vi "Left Find Data String (SubVI).vi"(11 "Sampled Data":string) -> (3 "Data String":string)   [LabVIEW 2015]
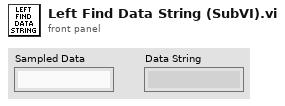
[diagram p1: front panel]
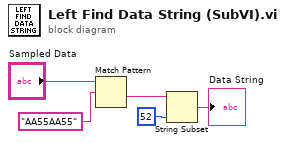
[diagram p0: block diagram]
diagram:
  n1 = Match Pattern(string="Sampled Data", regular expression="AA55AA55") -> (after substring=w2:string)  [unwired: 1 in, 3 out]
  n2 = String Subset(string=w2, length (rest)=52 ("length (rest)")) -> (substring=→"Data String":string)  [unwired: 1 in]
